vi "Receiver_Example - 2 Channel - Experiment_11.vi"() -> ()   [LabVIEW 2022 SP3]
uses:
  <vilib>/httpClient/LabVIEWHTTPClient.lvlib
panel:
  out "OutputHPCH0":i8[](array[numeric])
  out "HP - CH0 3":dbl format="%#_4g"
  out "HP - CH0 2":dbl format="%#_4g"
  out "BER 16QAM":dbl
  out "LP - CH0":dbl format="%#_4g"
  in  "url 2":string="http://Cobot280-02.local:5000"
  out "Numeric":i32
  out "HP - CH0":dbl format="%#_4g"
  in  "url":string="http://Cobot280-01.local:5000"
  out "x = 0?":bool
  out "iterationsIM":dbl
  in  "State":i32
  in  "Counter":dbl
  in  "Tab Control 3":enum32{"OFDM - 4QAM", "16QAM"}(tab)
  in  "Switch mode":bool
  in  "Tab Control":T1(tab)
  in  "USRP ControledParameters":T2={"Active Antenna"="RX2", "Gain (dB)"=10.0, "Carrier Frequency"=2400000000.0, "IQ Rate"=2000000.0, "Active channels"="0,1"} {"IQ Rate" format="%#_6p"; "Carrier Frequency" format="%#_6p"; "Gain (dB)" format="%#_6f"}
  in  "Device selection":refnum<k15>="RIO0"
  in  "Trigger level":dbl=0.005 format="%f"
  out "CH0":T3
  out "CH1":T3
  out "SIG valid? - CH1":bool
  out "SIG valid? - CH0":bool
  out "Frequency offset - CH1":dbl
  out "Frequency offset - CH0":dbl
  out "Coerced Parameters":T4={"IQ Rate"=100000.0, "Carrier  Freq."=100000.0, "Gain"=0.0} {"Gain" format="%#_6f"; "Carrier  Freq." format="%#_6p"; "IQ Rate" format="%#_6p"}
  out "Error out":errorcluster
  in  "Expected message LP - CH0":string="Non Critical Data\nNon Critical Data\nNon Critical Data\nNon Critical Data\nNon Critical Data"
  in  "Expected message - CH1":string="Critical Dataaaaa\nCritical Dataaaaa\nCritical Dataaaaa\nCritical Dataaaaa\nCritical Dataaaaa"
  out "Expected message LP Detected CH0":string="Non Critical Data\nNon Critical Data\nNon Critical Data\nNon Critical Data\nNon Critical Data"
  out "Expected message HP Detected CH1":string="Non Critical Data\nNon Critical Data\nNon Critical Data\nNon Critical Data\nNon Critical Data"
  in  "Boolean":bool
  in  "Boolean 3":bool
  out "Expected message HP Detected CH0":string="Non Critical Data\nNon Critical Data\nNon Critical Data\nNon Critical Data\nNon Critical Data"
  in  "Expected message HP - CH0":string="Critical Dataaaaa\nCritical Dataaaaa\nCritical Dataaaaa\nCritical Dataaaaa\nCritical Dataaaaa"
  in  "Boolean 2":bool
  out "Inst. BER HP - CH0":dbl format="%#_4g"
  out "Acc. BER HP - CH0":dbl format="%#_4g"
  out "Acum. Err HP - CH0":dbl
  out "No. Bits HP - CH0":dbl
  out "Acc. BER LP - CH0":dbl format="%#_4g"
  out "Inst. BER - CH1":dbl format="%#_4g"
  out "Inst. BER LP - CH0":dbl format="%#_4g"
  out "No. Bits - CH1":dbl
  out "No. Bits LP - CH0":dbl
  out "Acum. Err - CH1":dbl
  out "Acum. Err LP - CH0":dbl
  in  "Record BER":bool
  in  "Refresh Button":bool
  out "Acc. BER - CH1":dbl format="%#_4g"
  in  "High-Power Window Size":dbl=15.0 format="%#_6p"
  in  "Low-Power Window Size - CH0":dbl=15.0 format="%#_6p"
  in  "Threshold":dbl=10.0
  in  "Channel":bool
  in  "Expected message HP - CH0 2":string="Critical Dataaaaa\nCritical Dataaaaa\nCritical Dataaaaa\nCritical Dataaaaa\nCritical Dataaaaa\nNon Critical Data\nNon Critical Data\nNon Critical Data\nNon Critical Data\nNon Critical Data"
  in  "Tab Control 2":enum32{"1 Channel", "2 Channel"}(tab)
  in  "Save data 1 channel":bool
  out "Constellation Map 1 Channel":cdb[](graph)
  out "Low-Power BER - 1 Channel":dbl(graph)
  out "High-Power BER - 1 Channel":dbl(graph)
  out "High-Power Decoded message - 1 Channel":string
  out "Low-Power Decoded message - 1 Channel":string
  in  "Color Box":u32(colorbox)=11025761
  in  "Color Box 2":u32(colorbox)=7377308
  out "Low-Power Decoded message - CH0":string
  out "Decoded message - CH1":string
  out "Constellation Map 2 Channel":cluster{"Constellation":cdb[]}[](graph)
  out "Low-Power BER - CH0":dbl(graph)
  out "High-Power BER":T5(graph)
  out "High-Power Decoded message - CH0":string
  out "CH1 2":bool
  out "CH0 2":bool
  in  "Save data 2 channels":bool
  in  "Save data":bool
  out "Expected message  HP  Detected 2":string="Critical Dataaaaa\nCritical Dataaaaa\nCritical Dataaaaa\nCritical Dataaaaa\nCritical Dataaaaa"
  in  "Boolean 4":bool
  in  "High-Power Window Size 2":dbl=15.0 format="%#_6p"
  out "High-Power Instantaneous BER Graph 2":u8(slide) scale=0.0..100.0
  out "High-Power BER Graph 2":dbl(graph)
  out "No. Bits HP 2":dbl
  out "Acc. BER  HP 2":dbl format="%#_4g"
  out "Acum. Err HP 2":dbl
  out "Inst. BER HP 2":dbl format="%#_4g"
  in  "Expected message 2 HP 2":string="Critical Dataaaaa\nCritical Dataaaaa\nCritical Dataaaaa\nCritical Dataaaaa\nCritical Dataaaaa"
  out "High-Power Decoded Message 2":string
  in  "Record BER 2":bool
  out "Constellation Map 2":cdb[](graph)
  out "Frequency offset 2":dbl
  out "SIG valid? 2":bool
  in  "Refresh Button 2":bool
  out "Error out 2":errorcluster
  in  "error in (no error)":errorcluster
  # "OFDM Superposition Coded Receiver"
  # "Superposition coded\n(criticality-aware)"
  # "Single stream\n(criticality-agnostic)"
  # "1 Channel"
  # "2 Channel"
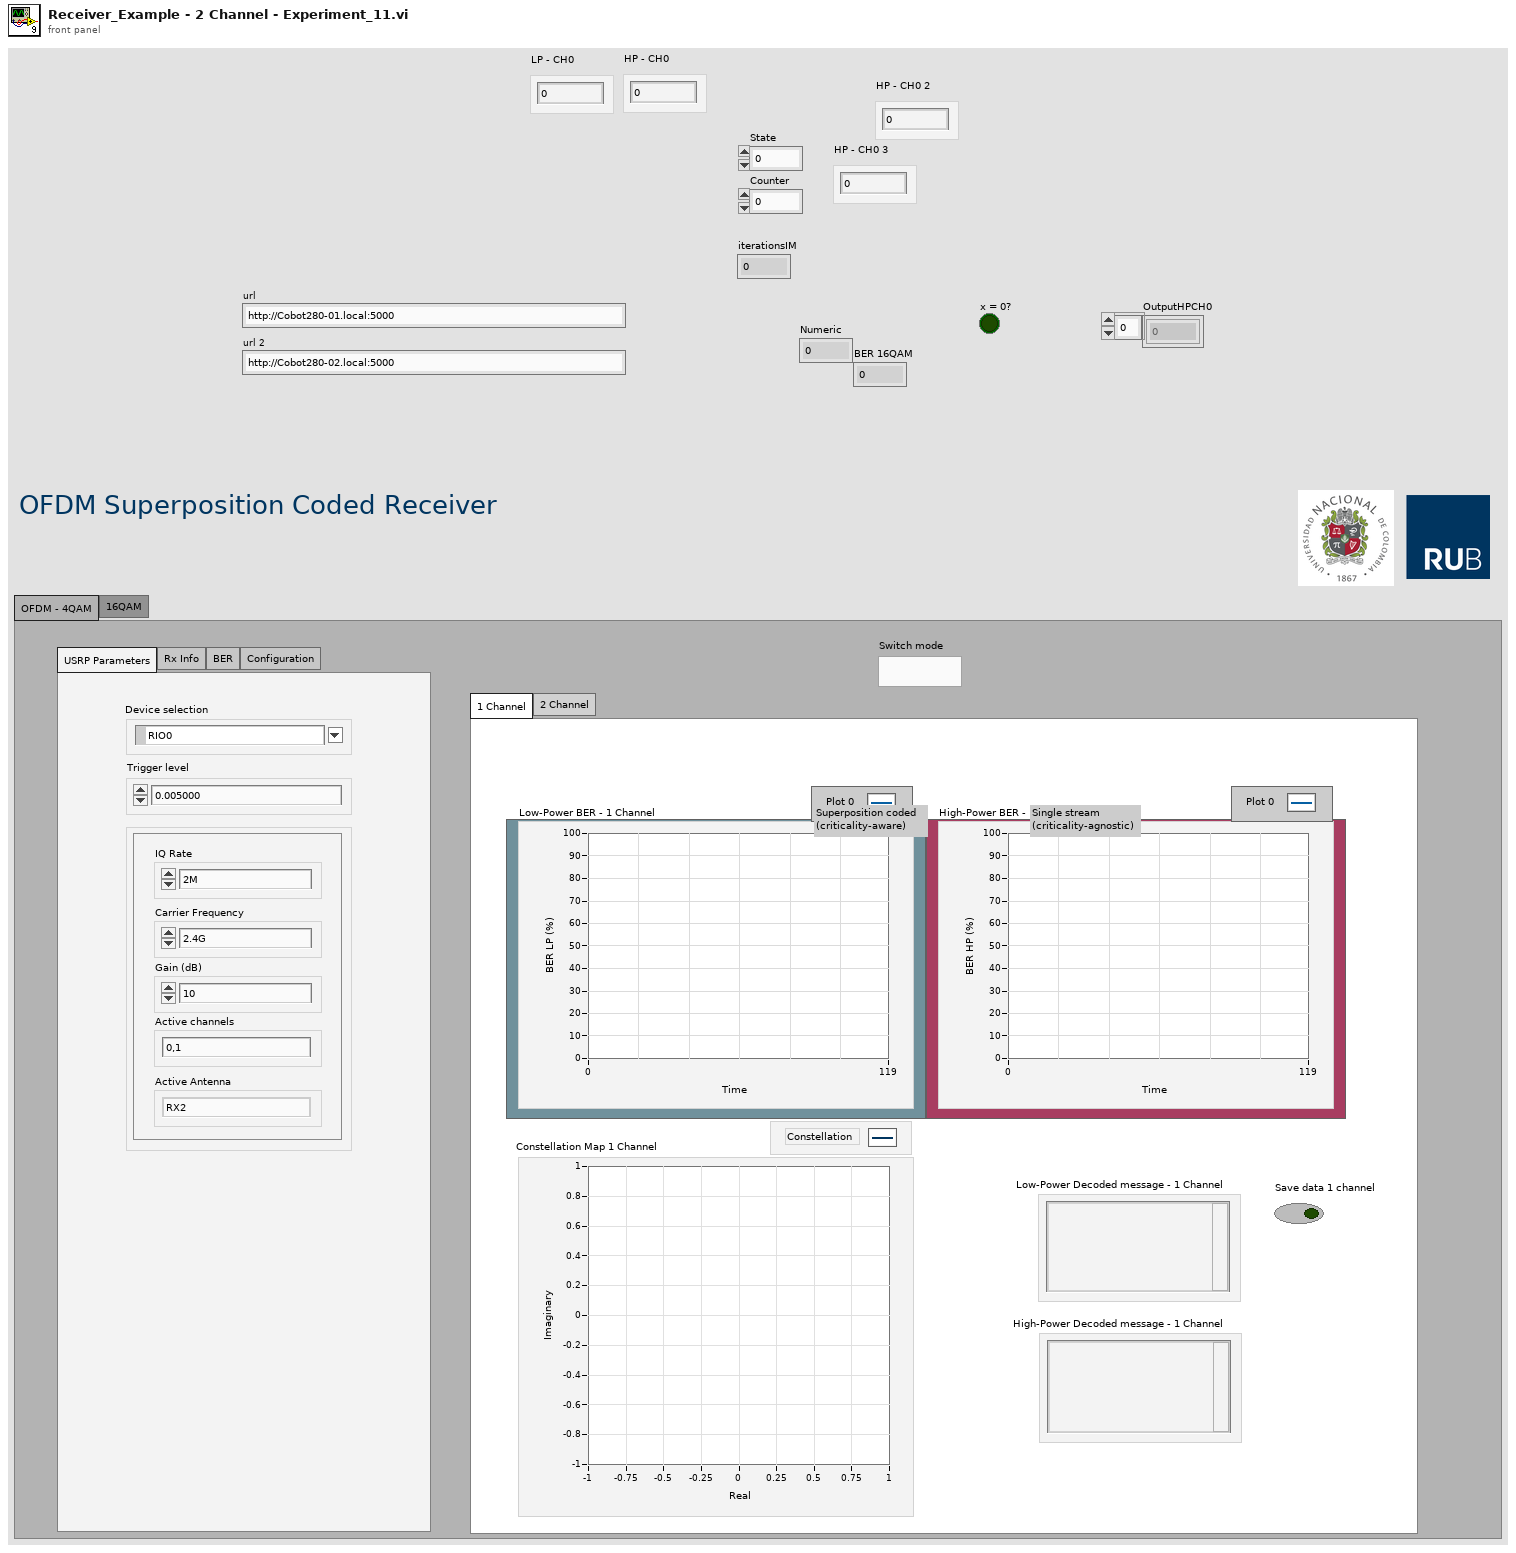
[diagram p1: front panel]
types:
  T1 = enum32{"USRP Parameters", "Rx Info", "BER", "Configuration"}
  T2 = cluster{"Active Antenna":string, "Gain (dB)":dbl, "Carrier Frequency":dbl, "IQ Rate":dbl, "Active channels":string}
  T3 = cluster{"Modulation type":enum16{"QPSK(4QAM)", "64QAM", "16QAM", "BPSK"}, "BCC rate (k/n)":enum16{"1/2", "2/3", "3/4"}}
  T4 = cluster{"IQ Rate":dbl, "Carrier  Freq.":dbl, "Gain":dbl}
  T5 = cluster{"Graph Instantaneous BER":dbl, "Graph Instantaneous BER":dbl, "Inst. BER - CH1":dbl}
  T6 = enum16{"open", "replace", "create", "open or create", "replace or create", "replace or create with confirmation"}
  T7 = cluster{"coerced IQ rate":dbl, "coerced carrier frequency":dbl, "coerced gain":dbl}
  T8 = cluster{"Graph Instantaneous BER":dbl, "Graph Instantaneous BER":dbl, "Graph Instantaneous BER":dbl}
  T9 = typedef "LabVIEWHTTPClient.lvlib/ClientHandle.ctl" = refnum<k1>
  T10 = typedef "angle_speed_def.ctl" = cluster{"degrees":dbl[], "speed":i32}
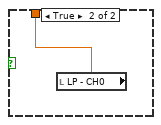
[diagram p2: hidden frame]
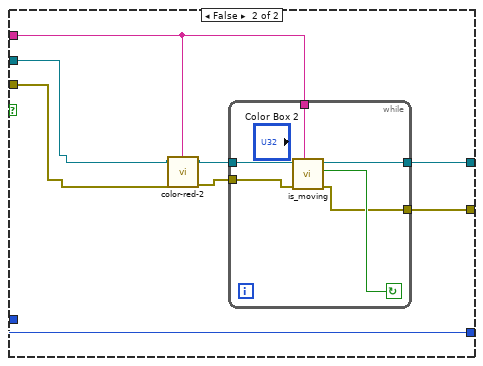
[diagram p3: hidden frame]
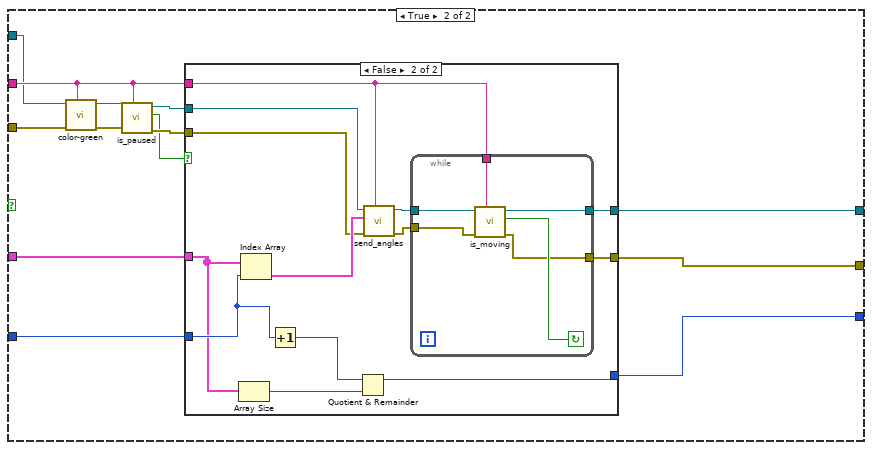
[diagram p4: hidden frame]
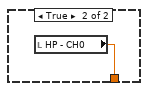
[diagram p6: hidden frame]
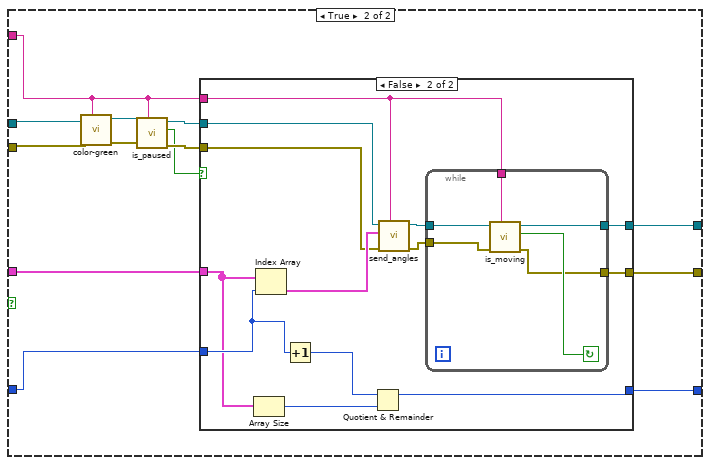
[diagram p8: hidden frame]
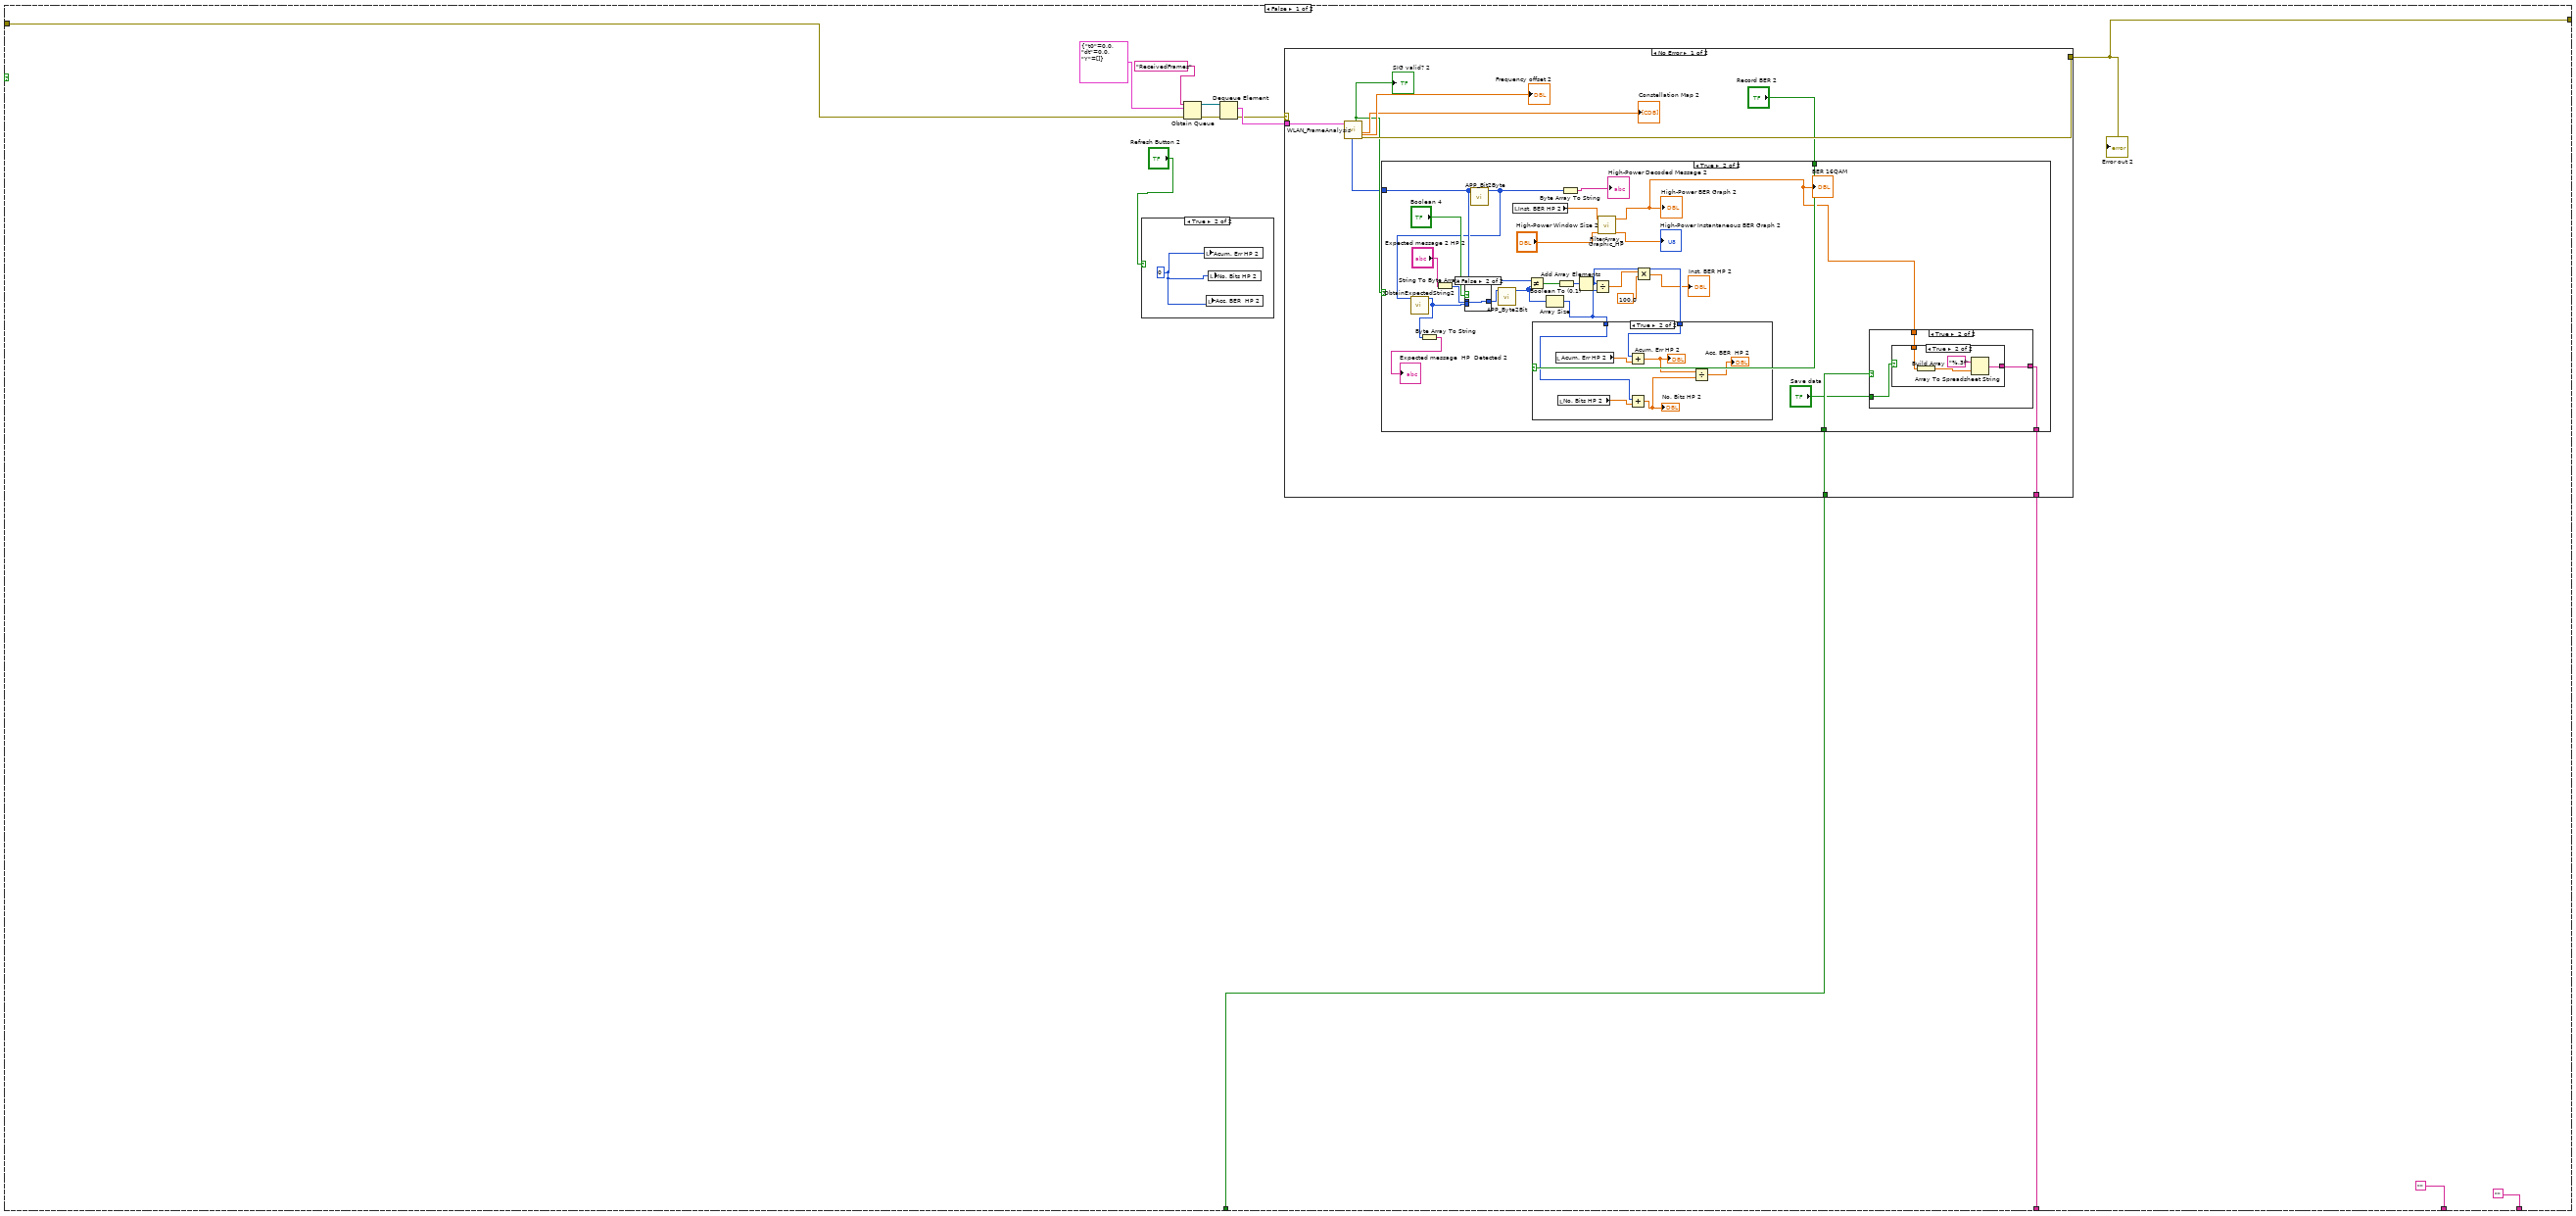
[diagram p10: hidden frame]
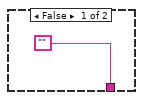
[diagram p12: hidden frame]
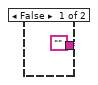
[diagram p13: hidden frame]
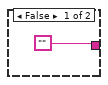
[diagram p14: hidden frame]
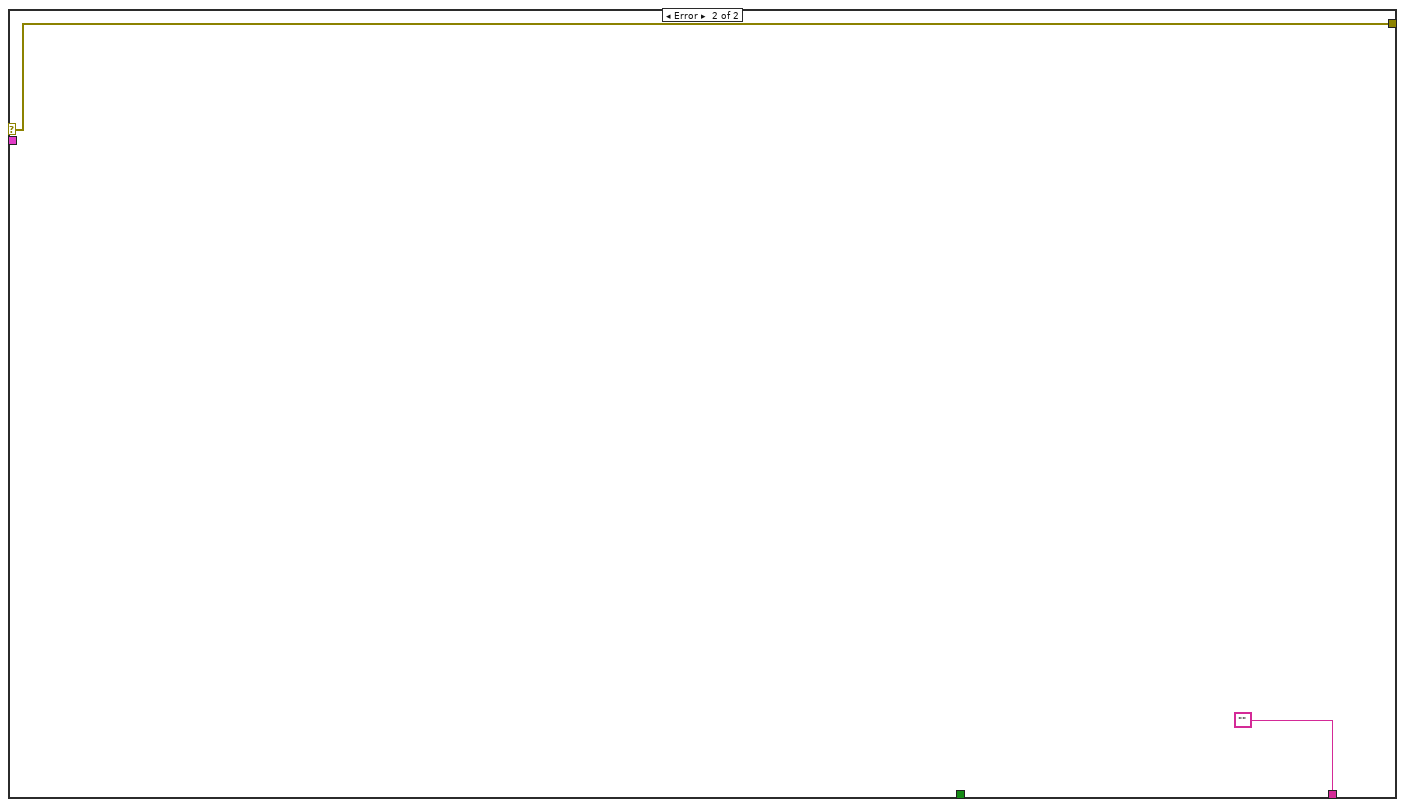
[diagram p17: hidden frame]
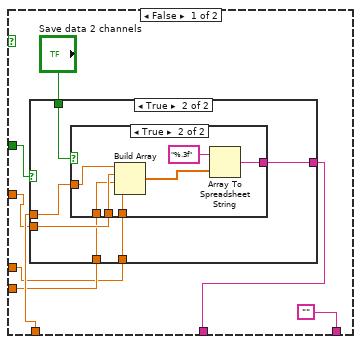
[diagram p19: hidden frame]
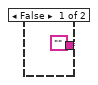
[diagram p20: hidden frame]
diagram:
  w23 = path "C:/Users/DKS/Desktop/Experiment/23_11_2023_with_graphs/12.10.2023/Supercoded Receiver with BER 12.10.2023/OFDM-Framework-LabVIEW-master/data"
  w45 = 0
  n1 = Build Path(base path=w23, name or relative path=path "data_OneChannel.txt" ("default name")) -> (appended path=w33:path)
  n2 = Build Path(base path=w23, name or relative path=path "data_16QAM.txt" ("default name")) -> (appended path=w43:path)
  n3 = Build Path(base path=w23, name or relative path=path "data_TwoChannels.txt" ("default name")) -> (appended path=w28:path)
  n4 = Delete(path (use dialog)=w33) -> (deleted path=w32:path)  [unwired: 4 in, 2 out]
  n5 = Delete(path (use dialog)=w43) -> (deleted path=w42:path)  [unwired: 4 in, 2 out]
  n6 = call "USRP_RXInit.vi"("device names"="Device selection", "USRP ControledParameters"="USRP ControledParameters", "error in (no error)"="error in (no error)") -> ("session handle out"=w48:refnum<k15>, "USRP CoercedParamters"=→"Coerced Parameters":T7, "error out"=w51:errorcluster)  [unwired: 5 in]
  n7 = Delete(path (use dialog)=w28) -> (deleted path=w27:path)  [unwired: 4 in, 2 out]
  n8 = Open/Create/Replace File(file path (use dialog)=w32, operation (0:open)=T6."create", access (0:read/write)=enum16{"read/write", "read-only", "write-only"}."write-only") -> (refnum out=w20:refnum<file>, error out=w19:errorcluster)  [unwired: 1 in, 3 out]
  n9 = Open/Create/Replace File(file path (use dialog)=w42, operation (0:open)=T6."create", access (0:read/write)=enum16{"read/write", "read-only", "write-only"}."write-only") -> (refnum out=w36:refnum<file>, error out=w37:errorcluster)  [unwired: 1 in, 3 out]
  n10 = Open/Create/Replace File(file path (use dialog)=w27, operation (0:open)=T6."create", access (0:read/write)=enum16{"read/write", "read-only", "write-only"}."write-only") -> (refnum out=w18:refnum<file>, error out=w17:errorcluster)  [unwired: 1 in, 3 out]
  n11 = call "WLAN_FrameCapture - 2 Channels.vi"("error in (no error)"=w51, "Trigger level"="Trigger level", "session handle"=w48) -> ()  [unwired: 8 in]
  n12 = while {
    tunnel: w51 -> [w77]
    tunnel: [w76] -> w49
    shift-right: [w71] -> w35
    shift-left: w37 -> [w69]
    shift-right: [w70] -> w34
    shift-left: w36 -> [w68]
    shift-right: [w65] -> w16
    shift-left: w20 -> [w66]
    shift-right: [w63] -> w15
    shift-left: w19 -> [w64]
    shift-right: [w59] -> w14
    shift-left: w18 -> [w62]
    shift-right: [w60] -> w13
    shift-left: w17 -> [w61]
    i -> [w56]
    stop <- FALSE stop-if-true
    n13 = Not(x="Switch mode") -> ()  [unwired: 1 out]
    n14 = Quotient & Remainder(x=w56, y=1) -> (x-y*floor(x/y)=w73:i32)  [unwired: 1 out]
    n15 = Equal To 0?(x=w73) -> (x = 0?=w72:bool)
    "x = 0?" <- w72
    n16 = case shown="True" TRUE {
      tunnel: w77 -> [w83 w164]
      tunnel: [w82 w163] -> w76
      tunnel: w72 -> [w81 w158]
      tunnel: [w80 ""] -> w67
      tunnel: ["" w157] -> w58
      tunnel: ["" w155] -> w57
      frame False {
        n17 = case shown="True" "Refresh Button 2" {
          frame False {
          }
          frame True {
            w91 = 0
            n18 = local write "Acum. Err HP 2"(w91) -> ()
            n19 = local write "Acc. BER  HP 2"(w91) -> ()
            n20 = local write "No. Bits HP 2"(w91) -> ()
          }
        }
        n21 = Obtain Queue(name (unnamed)="ReceivedFrames", element data type=cluster{"t0":dbl, "dt":dbl, "Y":cdb[]} {"t0"=0.0, "dt"=0.0, "Y"=[]} ("data"), error in (no error)=w83) -> (queue out=w84:refnum<queue>, error out=w87:errorcluster)  [unwired: 2 in, 1 out]
        n22 = Dequeue Element(queue=w84, error in (no error)=w87) -> (element=w86:cluster{"t0":dbl, "dt":dbl, "Y":cdb[]}, error out=w85:errorcluster)  [unwired: 1 in, 2 out]
        n23 = case shown="No Error" w85 {
          selector: w85 -> [_ w146]
          tunnel: w86 -> [w99 _]
          tunnel: [w100 w146] -> w82
          tunnel: w81 -> [w93 _]
          tunnel: [w92 ""] -> w80
          frame No Error {
            n24 = call "WLAN_FrameAnalysis.vi"("input cluster"=w99) -> ("error out"=w100:errorcluster, "Constellation"=→"Constellation Map 2":cdb[], "Frequency offset"=→"Frequency offset 2":dbl, "SIG valid?"=w95:bool, "outputbitsHP"=w94:i8[])  [unwired: 4 in, 2 out]
            "SIG valid? 2" <- w95
            n25 = case shown="True" w95 {
              tunnel: "Record BER 2" -> [_ w120]
              tunnel: w94 -> [_ w115]
              tunnel: w93 -> [_ w105]
              tunnel: ["" w103] -> w92
              frame False {
              }
              frame True {
                n26 = String To Byte Array(string="Expected message 2 HP 2") -> (unsigned byte array=w113:u8[])
                n27 = call "APP_Bit2Byte.vi"("input bit stream"=w115) -> ("output byte stream"=w109:u8[])  [unwired: 10 in]
                n28 = call "ObtainExpectedString2.vi"("Array"=w109) -> ("detectedMessage"=w111:i8[])  [unwired: 9 in]
                n29 = Byte Array To String(unsigned byte array=w111) -> (string=→"Expected message  HP  Detected 2":string)
                n30 = case shown="False" "Boolean 4" {
                  tunnel: [w136 w137] -> w114
                  tunnel: w113 -> [_ w137]
                  tunnel: w111 -> [w136 _]
                  frame True {
                  }
                  frame False {
                  }
                }
                n31 = call "APP_Byte2Bit.vi"("input byte stream"=w114) -> ("output bit stream"=w116:i8[])  [unwired: 10 in]
                n32 = local read "Inst. BER HP 2"() -> (w119:dbl)
                n33 = Not Equal?(x=w115, y=w116) -> (x != y?=w124:bool[])
                n34 = Array Size(array=w116) -> (size(s)=w121:i32)
                n35 = Boolean To (0,1)(Boolean=w124) -> (0, 1=w123:i16[])
                n36 = Byte Array To String(unsigned byte array=w109) -> (string=→"High-Power Decoded Message 2":string)
                n37 = Add Array Elements(numeric array=w123) -> (sum=w122:i16)
                n38 = case shown="True" w120 {
                  tunnel: w122 -> [_ w143]
                  tunnel: w121 -> [_ w138]
                  frame False {
                  }
                  frame True {
                    n39 = local read "Acum. Err HP 2"() -> (w144:dbl)
                    n40 = local read "No. Bits HP 2"() -> (w140:dbl)
                    n41 = Add(x=w143, y=w144) -> (x+y=w142:dbl)
                    "Acum. Err HP 2" <- w142
                    n42 = Add(x=w138, y=w140) -> (x+y=w139:dbl)
                    "No. Bits HP 2" <- w139
                    n43 = Divide(x=w142, y=w139) -> (x/y=→"Acc. BER  HP 2":dbl)
                  }
                }
                n44 = Divide(x=w122, y=w121) -> (x/y=w108:dbl)
                n45 = call "FilterArray_Graphic_HP.vi"("Window Size"="High-Power Window Size 2", "Instantaneous BER"=w119) -> ("Slide Bar"=→"High-Power Instantaneous BER Graph 2":dbl, "Graph Instantaneous BER"=w102:dbl)  [unwired: 4 in]
                "High-Power BER Graph 2" <- w102
                "BER 16QAM" <- w102
                n46 = Multiply(x=w108, y=100.0) -> (x*y=→"Inst. BER HP 2":dbl)
                n47 = case shown="True" w105 {
                  tunnel: ["" w130] -> w103
                  tunnel: w102 -> [_ w129]
                  tunnel: "Save data" -> [_ w128]
                  frame False {
                  }
                  frame True {
                    n48 = case shown="True" w128 {
                      tunnel: ["" w133] -> w130
                      tunnel: w129 -> [_ w132]
                      frame False {
                      }
                      frame True {
                        n49 = Build Array(w132) -> (w135:dbl[])
                        n50 = Array To Spreadsheet String(array=w135, 3:"%.3f") -> (spreadsheet string=w133:string)  [unwired: 1 out]
                      }
                    }
                  }
                }
              }
            }
          }
          frame Error {
          }
        }
        "Error out 2" <- w82
      }
      frame True {
        w200 = cluster{"t0":dbl, "dt":dbl, "Y":cdb[]} {"t0"=0.0, "dt"=0.0, "Y"=[]} ("data")
        n51 = Obtain Queue(name (unnamed)="ReceivedFrames", element data type=w200, error in (no error)=w164) -> (queue out=w165:refnum<queue>, error out=w167:errorcluster)  [unwired: 2 in, 1 out]
        n52 = Obtain Queue(name (unnamed)="ReceivedFrames_1", element data type=w200, error in (no error)=w164) -> (queue out=w169:refnum<queue>, error out=w170:errorcluster)  [unwired: 2 in, 1 out]
        n53 = Dequeue Element(queue=w165, error in (no error)=w167) -> (element=w166:cluster{"t0":dbl, "dt":dbl, "Y":cdb[]}, error out=w173:errorcluster)  [unwired: 1 in, 2 out]
        n54 = Dequeue Element(queue=w169, error in (no error)=w170) -> (element=w175:cluster{"t0":dbl, "dt":dbl, "Y":cdb[]}, error out=w179:errorcluster)  [unwired: 1 in, 2 out]
        n55 = Not(x="Channel") -> (.not. x?=w159:bool)
        n56 = Merge Errors(w173, w179) -> (w172:errorcluster)
        n57 = case shown="No Error" w172 {
          tunnel: w166 -> [w349 _]
          tunnel: w172 -> [_ w449]
          tunnel: w173 -> [w346 _]
          tunnel: [w345 dbl[] []] -> w191
          tunnel: [w344 w449] -> w176
          tunnel: "Record BER" -> [w343 _]
          tunnel: "Record BER" -> [w342 _]
          tunnel: w159 -> [w341 _]
          frame No Error {
            n58 = local read "Switch mode"() -> (w340:bool)
            n59 = call "WLAN_FrameAnalysis.vi"("error in (no error)"=w346, "input cluster"=w349) -> ("error out"=w344:errorcluster, "Constellation"=w345:cdb[], "Modulation parameter"=w350:T3, "output bits"=w351:i8[], "Frequency offset"=→"Frequency offset - CH0":dbl, "SIG valid?"=w347:bool, "outputbitsHP"=w348:i8[])  [unwired: 3 in]
            "SIG valid? - CH0" <- w347
            n60 = Not(x=w340) -> (.not. x?=w339:bool)
            n61 = case shown="True" w347 {
              tunnel: w351 -> [_ w401]
              tunnel: w350 -> [_ w424]
              tunnel: w342 -> [_ w420]
              tunnel: w341 -> [_ w404]
              tunnel: w339 -> [_ w402]
              frame False {
              }
              frame True {
                n62 = case shown="False" w402 {
                  tunnel: w401 -> [_ w434]
                  tunnel: [w432 w434] -> w403
                  frame False {
                    n63 = local read "OutputHPCH0"() -> (w431:i8[])
                    n64 = Array Size(array=w431) -> (size(s)=w430:i32)
                    n65 = Divide(x=w430, y=2) -> (x/y=w427:dbl)
                    n66 = Add(x=4.0, y=w427) -> (x+y=w429:dbl)
                    n67 = Subtract(x=w427, y=5.0) -> (x-y=w425:dbl)
                    n68 = Array Subset(array=w431, index=w429, length=w425) -> (w432:i8[])
                  }
                  frame True {
                  }
                }
                n69 = String To Byte Array(string="Expected message LP - CH0") -> (unsigned byte array=w413:u8[])
                n70 = call "APP_Bit2Byte.vi"("input bit stream"=w403) -> ("output byte stream"=w412:u8[])  [unwired: 10 in]
                n71 = call "ObtainExpectedString.vi"("Array"=w412) -> ("detectedMessage"=w409:i8[])  [unwired: 9 in]
                n72 = Byte Array To String(unsigned byte array=w409) -> (string=→"Expected message LP Detected CH0":string)
                n73 = case shown="False" "Boolean" {
                  tunnel: [w439 w440] -> w415
                  tunnel: w413 -> [_ w440]
                  tunnel: w409 -> [w439 _]
                  frame True {
                  }
                  frame False {
                  }
                }
                n74 = call "APP_Byte2Bit.vi"("input byte stream"=w415) -> ("output bit stream"=w414:i8[])  [unwired: 10 in]
                n75 = Not Equal?(x=w401, y=w414) -> (x != y?=w422:bool[])
                n76 = Array Size(array=w414) -> (size(s)=w419:i32)
                n77 = Boolean To (0,1)(Boolean=w422) -> (0, 1=w423:i16[])
                n78 = Add Array Elements(numeric array=w423) -> (sum=w418:i16)
                n79 = case shown="True" w420 {
                  tunnel: w419 -> [_ w446]
                  tunnel: w418 -> [_ w444]
                  frame False {
                  }
                  frame True {
                    n80 = local read "Acum. Err LP - CH0"() -> (w445:dbl)
                    n81 = local read "No. Bits LP - CH0"() -> (w447:dbl)
                    n82 = Add(x=w446, y=w447) -> (x+y=w443:dbl)
                    n83 = Add(x=w444, y=w445) -> (x+y=w442:dbl)
                    "Acum. Err LP - CH0" <- w442
                    n84 = local write "No. Bits LP - CH0"(w443) -> ()
                    n85 = Divide(x=w442, y=w443) -> (x/y=→"Acc. BER LP - CH0":dbl)
                  }
                }
                n86 = Divide(x=w418, y=w419) -> (x/y=w417:dbl)
                n87 = Multiply(x=w417, y=100.0) -> (x*y=→"Inst. BER LP - CH0":dbl)
                n88 = Byte Array To String(unsigned byte array=w412) -> (string=w407:string)
                n89 = case shown="True" w404 {
                  tunnel: w407 -> [w436 w438]
                  tunnel: ["" ("string") w438] -> w406
                  tunnel: [w436 "" ("string")] -> w405
                  frame False {
                  }
                  frame True {
                  }
                }
                "Low-Power Decoded message - CH0" <- w405
                "Low-Power Decoded message - 1 Channel" <- w406
                "CH0" <- w424
              }
            }
            n90 = case shown="True" w347 {
              tunnel: w348 -> [_ w354]
              tunnel: w343 -> [_ w372]
              tunnel: w341 -> [_ w359]
              tunnel: w339 -> [_ w357]
              frame False {
              }
              frame True {
                n91 = String To Byte Array(string="Expected message HP - CH0") -> (unsigned byte array=w356:u8[])
                n92 = case shown="False" w357 {
                  tunnel: w354 -> [w383 w387]
                  tunnel: [w384 w387] -> w358
                  tunnel: [w376 w386] -> w353
                  tunnel: w356 -> [_ w386]
                  frame False {
                    n93 = Array Size(array=w383) -> (size(s)=w380:i32)
                    n94 = Divide(x=w380, y=2) -> (x/y=w379:dbl)
                    n95 = Subtract(x=w379, y=5) -> (x-y=w381:dbl)
                    n96 = Array Subset(array=w383, index=0, length=w381) -> (w384:i8[])
                    n97 = String To Byte Array(string="Expected message HP - CH0 2") -> (unsigned byte array=w376:u8[])
                  }
                  frame True {
                  }
                }
                n98 = call "APP_Byte2Bit.vi"("input byte stream"=w353) -> ("output bit stream"=w355:i8[])  [unwired: 10 in]
                n99 = Not Equal?(x=w354, y=w355) -> (x != y?=w374:bool[])
                n100 = Array Size(array=w355) -> (size(s)=w371:i32)
                n101 = Boolean To (0,1)(Boolean=w374) -> (0, 1=w375:i16[])
                n102 = Add Array Elements(numeric array=w375) -> (sum=w370:i16)
                n103 = case shown="True" w372 {
                  tunnel: w371 -> [_ w399]
                  tunnel: w370 -> [_ w397]
                  frame False {
                  }
                  frame True {
                    n104 = local read "Acum. Err HP - CH0"() -> (w398:dbl)
                    n105 = local read "No. Bits HP - CH0"() -> (w400:dbl)
                    n106 = Add(x=w399, y=w400) -> (x+y=w396:dbl)
                    n107 = local write "No. Bits HP - CH0"(w396) -> ()
                    n108 = Add(x=w397, y=w398) -> (x+y=w395:dbl)
                    "Acum. Err HP - CH0" <- w395
                    n109 = Divide(x=w395, y=w396) -> (x/y=→"Acc. BER HP - CH0":dbl)
                  }
                }
                n110 = Divide(x=w370, y=w371) -> (x/y=w369:dbl)
                n111 = call "APP_Bit2Byte.vi"("input bit stream"=w358) -> ("output byte stream"=w365:u8[])  [unwired: 10 in]
                n112 = call "ObtainExpectedString2.vi"("Array"=w365) -> ("detectedMessage"=w364:i8[])  [unwired: 9 in]
                n113 = Byte Array To String(unsigned byte array=w364) -> (string=→"Expected message HP Detected CH0":string)
                n114 = case shown="False" "Boolean 2" {
                  tunnel: [w392 w393] -> _
                  tunnel: w356 -> [_ w393]
                  tunnel: w364 -> [w392 _]
                  frame True {
                  }
                  frame False {
                  }
                }
                n115 = Multiply(x=w369, y=100.0) -> (x*y=→"Inst. BER HP - CH0":dbl)
                n116 = Byte Array To String(unsigned byte array=w365) -> (string=w360:string)
                n117 = case shown="False" w359 {
                  tunnel: w360 -> [w389 w391]
                  tunnel: ["" ("string") w391] -> w361
                  tunnel: [w389 "" ("string")] -> w362
                  frame False {
                  }
                  frame True {
                  }
                }
                "High-Power Decoded message - CH0" <- w362
                "High-Power Decoded message - 1 Channel" <- w361
                "OutputHPCH0" <- w354
              }
            }
          }
          frame Error {
          }
        }
        n118 = case shown="No Error" w179 {
          tunnel: w175 -> [w299 _]
          tunnel: "Record BER" -> [w297 _]
          tunnel: [w296 w338] -> w177
          tunnel: [w295 dbl[] []] -> w178
          tunnel: w179 -> [w294 w338]
          tunnel: w159 -> [w293 _]
          frame No Error {
            n119 = call "WLAN_FrameAnalysis.vi"("error in (no error)"=w294, "input cluster"=w299) -> ("error out"=w296:errorcluster, "Constellation"=w295:cdb[], "Modulation parameter"=w302:T3, "Frequency offset"=→"Frequency offset - CH1":dbl, "SIG valid?"=w298:bool, "outputbitsHP"=w300:i8[])  [unwired: 3 in, 1 out]
            "SIG valid? - CH1" <- w298
            n120 = case shown="True" "Refresh Button" {
              frame False {
              }
              frame True {
                w304 = 0
                n121 = local write "Acum. Err HP - CH0"(w304) -> ()
                n122 = local write "Acc. BER HP - CH0"(w304) -> ()
                n123 = local write "Acum. Err LP - CH0"(w304) -> ()
                n124 = local write "No. Bits LP - CH0"(w304) -> ()
                n125 = local write "No. Bits HP - CH0"(w304) -> ()
                n126 = local write "Acc. BER LP - CH0"(w304) -> ()
                n127 = local write "Acum. Err - CH1"(w304) -> ()
                n128 = local write "No. Bits - CH1"(w304) -> ()
                n129 = local write "Acc. BER - CH1"(w304) -> ()
              }
            }
            n130 = case shown="True" w298 {
              tunnel: w300 -> [_ w311]
              tunnel: w302 -> [_ w325]
              tunnel: w297 -> [_ w308]
              tunnel: w293 -> [_ w305]
              frame False {
              }
              frame True {
                n131 = call "APP_Bit2Byte.vi"("input bit stream"=w311) -> ("output byte stream"=w314:u8[])  [unwired: 10 in]
                n132 = call "ObtainExpectedString3.vi"("Array"=w314) -> ("detectedMessage"=w313:i8[])  [unwired: 9 in]
                n133 = Byte Array To String(unsigned byte array=w314) -> (string=w306:string)
                n134 = String To Byte Array(string="Expected message - CH1") -> (unsigned byte array=w315:u8[])
                n135 = Byte Array To String(unsigned byte array=w313) -> (string=→"Expected message HP Detected CH1":string)
                n136 = case shown="False" "Boolean 3" {
                  tunnel: [w328 w329] -> w317
                  tunnel: w315 -> [_ w329]
                  tunnel: w313 -> [w328 _]
                  frame True {
                  }
                  frame False {
                  }
                }
                n137 = call "APP_Byte2Bit.vi"("input byte stream"=w317) -> ("output bit stream"=w316:i8[])  [unwired: 10 in]
                n138 = Not Equal?(x=w311, y=w316) -> (x != y?=w323:bool[])
                n139 = Array Size(array=w316) -> (size(s)=w321:i32)
                n140 = Boolean To (0,1)(Boolean=w323) -> (0, 1=w324:i16[])
                n141 = Add Array Elements(numeric array=w324) -> (sum=w320:i16)
                n142 = case shown="True" w308 {
                  tunnel: w321 -> [_ w335]
                  tunnel: w320 -> [_ w333]
                  frame False {
                  }
                  frame True {
                    n143 = local read "No. Bits - CH1"() -> (w336:dbl)
                    n144 = local read "Acum. Err - CH1"() -> (w334:dbl)
                    n145 = Add(x=w335, y=w336) -> (x+y=w332:dbl)
                    n146 = Add(x=w333, y=w334) -> (x+y=w331:dbl)
                    "Acum. Err - CH1" <- w331
                    n147 = local write "No. Bits - CH1"(w332) -> ()
                    n148 = Divide(x=w331, y=w332) -> (x/y=→"Acc. BER - CH1":dbl)
                  }
                }
                n149 = case shown="True" w305 {
                  tunnel: w306 -> [w326 _]
                  tunnel: [w326 "" ("string")] -> w307
                  frame False {
                  }
                  frame True {
                  }
                }
                "Decoded message - CH1" <- w307
                n150 = Divide(x=w320, y=w321) -> (x/y=w318:dbl)
                n151 = Multiply(x=w318, y=100.0) -> (x*y=→"Inst. BER - CH1":dbl)
                "CH1" <- w325
              }
            }
          }
          frame Error {
          }
        }
        n152 = local read "Inst. BER HP - CH0"() -> (w196:dbl)
        n153 = local read "Inst. BER - CH1"() -> (w186:dbl)
        n154 = Bundle("Constellation"=w191) -> (w190:cluster{"Constellation":cdb[]})  [unwired: 1 in]
        n155 = Bundle("Constellation"=w178) -> (w174:cluster{"Constellation":cdb[]})  [unwired: 1 in]
        n156 = local read "Inst. BER LP - CH0"() -> (w161:dbl)
        n157 = Merge Errors(w176, w177) -> (w163:errorcluster)
        "Error out" <- w163
        n158 = Build Array(w190, w174) -> (w193:cluster{"Constellation":cdb[]}[])
        n159 = call "FilterArray_Graphic_CH1.vi"("Window Size"="High-Power Window Size", "Instantaneous BER"=w186) -> ("Graph Instantaneous BER"=w156:dbl)  [unwired: 4 in, 1 out]
        n160 = call "FilterArray_Graphic_HP.vi"("Window Size"="High-Power Window Size", "Instantaneous BER"=w196) -> ("Graph Instantaneous BER"=w153:dbl)  [unwired: 4 in, 1 out]
        "HP - CH0" <- w153
        n161 = case shown="0, Default" "State" {
          tunnel: "Counter" -> [w261 w281]
          tunnel: [w268 w284] -> w182
          tunnel: "Counter" -> [w256 w274]
          tunnel: [w265 w283] -> w183
          tunnel: [w263 w282] -> w154
          tunnel: w153 -> [w262 w279]
          tunnel: w156 -> [w260 w280]
          tunnel: 10.0 ("y") -> [w259 w275]
          frame 0, Default {
            n162 = Greater?(x=w262, y=10.0) -> (0:w269:bool)
            n163 = Equal?(x=w256, y=w259) -> (x = y?=w264:bool)
            n164 = Add(x=w261, y=1.0) -> (x+y=w271:dbl)
            n165 = Greater?(x=w256, y=w259) -> (0:w258:bool)
            n166 = Select(t=w271, s=w269, f=0.0) -> (s? t:f=w268:dbl)
            n167 = Select(t=w260, s=w264, f=w262) -> (s? t:f=w263:dbl)
            n168 = Select(t=1.0, s=w264, f=0.0) -> (s? t:f=w265:dbl)
            n169 = Select(t=0.0, s=w258, f=w256) -> (s? t:f=w255:dbl)
            n170 = local write "Counter"(w255) -> ()
          }
          frame 1 {
            n171 = Less?(x=w279, y=10.0) -> (x < y?=w285:bool)
            n172 = Greater?(x=w274, y=w275) -> (0:w277:bool)
            n173 = Equal?(x=w274, y=w275) -> (x = y?=w287:bool)
            n174 = Add(x=w281, y=1.0) -> (x+y=w291:dbl)
            n175 = Select(t=w291, s=w285, f=0.0) -> (s? t:f=w284:dbl)
            n176 = Select(t=0.0, s=w277, f=w274) -> (s? t:f=w278:dbl)
            n177 = local write "Counter"(w278) -> ()
            n178 = Select(t=w279, s=w287, f=w280) -> (s? t:f=w282:dbl)
            n179 = Select(t=0.0, s=w287, f=1.0) -> (s? t:f=w283:dbl)
          }
        }
        n180 = call "FilterArray_Graphic_LP.vi"("Window Size"="Low-Power Window Size - CH0", "Instantaneous BER"=w161) -> ("Graph Instantaneous BER"=w152:dbl)  [unwired: 4 in, 1 out]
        "LP - CH0" <- w152
        n181 = case shown="True" w159 {
          tunnel: [cdb[] [] ("Constellation") w254] -> w192
          tunnel: w191 -> [_ w254]
          tunnel: w193 -> [w252 _]
          tunnel: [w252 cluster{"Constellation":cdb[]}[] []] -> w194
          frame False {
          }
          frame True {
          }
        }
        "Constellation Map 2 Channel" <- w194
        "Constellation Map 1 Channel" <- w192
        n182 = local read "Switch mode"() -> (w151:bool)
        n183 = case shown="False" w159 {
          tunnel: w152 -> [w244 w246]
          tunnel: [nan ("Graph Instantaneous BER") w246] -> w148
          tunnel: [w244 nan ("Graph Instantaneous BER")] -> w149
          frame False {
          }
          frame True {
          }
        }
        "Low-Power BER - CH0" <- w149
        n184 = Bundle("Graph Instantaneous BER"=w153, "Graph Instantaneous BER"=w156, "Graph Instantaneous BER"=w154) -> (w198:T8)  [unwired: 1 in]
        n185 = Equal To 0?(x="State") -> (x = 0?=w189:bool)
        "CH0 2" <- w189
        n186 = Not(x=w151) -> (.not. x?=w150:bool)
        n187 = Not(x=w189) -> (.not. x?=→"CH1 2":bool)
        n188 = case shown="False" w159 {
          tunnel: w153 -> [_ w250]
          tunnel: [nan w250] -> w197
          tunnel: w198 -> [w248 _]
          tunnel: [w248 T8 {"Graph Instantaneous BER"=nan, "Graph Instantaneous BER"=nan, "Graph Instantaneous BER"=nan}] -> w199
          frame False {
          }
          frame True {
          }
        }
        "High-Power BER" <- w199
        "High-Power BER - 1 Channel" <- w197
        n189 = case shown="False" w150 {
          tunnel: w148 -> [_ w202]
          tunnel: [w201 w202] -> w147
          frame False {
            n190 = local read "HP - CH0"() -> (w201:dbl)
          }
          frame True {
          }
        }
        "Low-Power BER - 1 Channel" <- w147
        n191 = local write "Counter"(w182) -> ()
        n192 = local write "State"(w183) -> ()
        n193 = case shown="True" w159 {
          tunnel: w152 -> [w207 w231]
          tunnel: w153 -> [w206 w230]
          tunnel: w158 -> [w209 w229]
          tunnel: ["" w227] -> w157
          tunnel: w156 -> [w205 _]
          tunnel: w154 -> [w204 _]
          tunnel: [w203 ""] -> w155
          frame False {
            n194 = case shown="True" w209 {
              tunnel: ["" w217] -> w203
              tunnel: w207 -> [_ w215]
              tunnel: w206 -> [_ w216]
              tunnel: "Save data 2 channels" -> [_ w214]
              tunnel: w205 -> [_ w213]
              tunnel: w204 -> [_ w212]
              frame False {
              }
              frame True {
                n195 = case shown="True" w214 {
                  tunnel: ["" w223] -> w217
                  tunnel: w215 -> [_ w222]
                  tunnel: w216 -> [_ w221]
                  tunnel: w213 -> [_ w220]
                  tunnel: w212 -> [_ w219]
                  frame False {
                  }
                  frame True {
                    n196 = Build Array(w222, w221, w220, w219) -> (w225:dbl[])
                    n197 = Array To Spreadsheet String(array=w225, 3:"%.3f") -> (spreadsheet string=w223:string)  [unwired: 1 out]
                  }
                }
              }
            }
          }
          frame True {
            n198 = case shown="True" w229 {
              tunnel: ["" w236] -> w227
              tunnel: w231 -> [_ w234]
              tunnel: w230 -> [_ w235]
              tunnel: "Save data 1 channel" -> [_ w233]
              frame False {
              }
              frame True {
                n199 = case shown="True" w233 {
                  tunnel: ["" w240] -> w236
                  tunnel: w234 -> [_ w239]
                  tunnel: w235 -> [_ w238]
                  frame False {
                  }
                  frame True {
                    n200 = Build Array(w239, w238) -> (w242:dbl[])
                    n201 = Array To Spreadsheet String(array=w242, 3:"%.3f") -> (spreadsheet string=w240:string)  [unwired: 1 out]
                  }
                }
              }
            }
          }
        }
      }
    }
    n202 = Write to Text File(file (use dialog)=w62, text=w57, error in=w61) -> (refnum out=w59:refnum<file>, error out=w60:errorcluster)  [unwired: 1 in, 1 out]
    n203 = Write to Text File(file (use dialog)=w68, text=w67, error in=w69) -> (refnum out=w70:refnum<file>, error out=w71:errorcluster)  [unwired: 1 in, 1 out]
    n204 = Write to Text File(file (use dialog)=w66, text=w58, error in=w64) -> (refnum out=w65:refnum<file>, error out=w63:errorcluster)  [unwired: 1 in, 1 out]
    "Numeric" <- w56
  }
  n205 = call <vilib>:"OpenHandle.vi"() -> ("client handle out"=w7:T9, "error out"=w8:errorcluster)  [unwired: 14 in]
  n206 = call "wave.vi"() -> ("sequenz"=w9:T10[])  [unwired: 11 in]
  n207 = call <vilib>:"OpenHandle.vi"() -> ("client handle out"=w3:T9, "error out"=w2:errorcluster)  [unwired: 14 in]
  n208 = while {
    shift-right: [w459] -> _
    shift-left: 0 -> [w460]
    tunnel: w9 -> [w458]
    tunnel: w2 -> [w457]
    tunnel: w3 -> [w456]
    tunnel: [w455] -> w6
    tunnel: [w454] -> w4
    tunnel: "Threshold" -> [w453]
    stop <- FALSE stop-if-true
    n209 = local read "Switch mode"() -> (w451:bool)
    n210 = Not(x=w451) -> (.not. x?=w450:bool)
    n211 = case shown="False" w450 {
      tunnel: [w465 w466] -> w452
      frame False {
        n212 = local read "HP - CH0"() -> (w465:dbl)
      }
      frame True {
        n213 = local read "LP - CH0"() -> (w466:dbl)
      }
    }
    n214 = Wait (ms)(milliseconds to wait=u32 300) -> ()  [unwired: 1 out]
    n215 = Less?(x=w452, y=w453) -> (x < y?=w462:bool)
    n216 = case shown="False" w462 {
      tunnel: "url 2" -> [w471 w501]
      tunnel: w460 -> [w473 w500]
      tunnel: [w472 w499] -> w459
      tunnel: w458 -> [_ w498]
      tunnel: w457 -> [w468 w497]
      tunnel: w456 -> [w467 w496]
      tunnel: [w470 w495] -> w455
      tunnel: [w469 w494] -> w454
      frame False {
        n217 = call "is_paused.vi"("url"=w471, "error in (no error)"=w468, "client handle"=w467) -> ("error out"=w475:errorcluster, "paused"=w474:bool, "client handle out"=w476:T9)  [unwired: 6 in]
        n218 = case shown="True" w474 {
          tunnel: w471 -> [_ w482]
          tunnel: w475 -> [w478 w484]
          tunnel: w476 -> [w479 w483]
          tunnel: [w479 w487] -> w470
          tunnel: [w478 w486] -> w469
          tunnel: w473 -> [w477 w485]
          tunnel: [w477 w485] -> w472
          frame True {
          }
          frame False {
            n219 = call "color-red-2.vi"("url"=w482, "error in (no error)"=w484, "client handle"=w483) -> ("error out"=w480:errorcluster, "client handle out"=w481:T9)  [unwired: 7 in]
            n220 = while {
              tunnel: w482 -> [w493]
              tunnel: w481 -> [w492]
              tunnel: w480 -> [w491]
              tunnel: [w489] -> w487
              tunnel: [w488] -> w486
              stop <- w490 continue-if-true
              n221 = call "is_moving.vi"("string"=w493, "error in (no error)"=w491, "client handle"=w492) -> ("error out"=w488:errorcluster, "moving"=w490:bool, "client handle out"=w489:T9)  [unwired: 6 in]
            }
          }
        }
      }
      frame True {
        n222 = call "color-green.vi"("url"=w501, "error in (no error)"=w497, "client handle"=w496) -> ("error out"=w503:errorcluster, "client handle out"=w502:T9)  [unwired: 7 in]
        n223 = call "is_paused.vi"("url"=w501, "error in (no error)"=w503, "client handle"=w502) -> ("error out"=w505:errorcluster, "paused"=w504:bool, "client handle out"=w506:T9)  [unwired: 6 in]
        n224 = case shown="False" w504 {
          tunnel: w498 -> [_ w514]
          tunnel: w500 -> [w507 w516]
          tunnel: w501 -> [_ w519]
          tunnel: w505 -> [w508 w521]
          tunnel: w506 -> [w509 w520]
          tunnel: [w507 w512] -> w499
          tunnel: [w509 w511] -> w495
          tunnel: [w508 w510] -> w494
          frame True {
          }
          frame False {
            n225 = Array Size(array=w514) -> (size(s)=w513:i32)
            n226 = Index Array(array=w514, index=w516) -> (element=w522:T10)
            n227 = Increment(x=w516) -> (x+1=w515:i32)
            n228 = Quotient & Remainder(x=w515, y=w513) -> (x-y*floor(x/y)=w512:i32)  [unwired: 1 out]
            n229 = call "send_angles.vi"("url"=w519, "error in (no error)"=w521, "angles and speed"=w522, "client handle"=w520) -> ("error out"=w517:errorcluster, "client handle out"=w518:T9)  [unwired: 6 in]
            n230 = while {
              tunnel: w519 -> [w528]
              tunnel: w518 -> [w527]
              tunnel: w517 -> [w526]
              tunnel: [w524] -> w511
              tunnel: [w523] -> w510
              stop <- w525 continue-if-true
              n231 = call "is_moving.vi"("string"=w528, "error in (no error)"=w526, "client handle"=w527) -> ("error out"=w523:errorcluster, "moving"=w525:bool, "client handle out"=w524:T9)  [unwired: 6 in]
            }
          }
        }
      }
    }
  }
  n232 = while {
    tunnel: w9 -> [w542]
    tunnel: w8 -> [w541]
    tunnel: w7 -> [w540]
    tunnel: [w539] -> w12
    tunnel: [w538] -> w5
    shift-right: [w536] -> _
    shift-left: 0 -> [w537]
    tunnel: "Threshold" -> [w531]
    stop <- FALSE stop-if-true
    n233 = local read "Switch mode"() -> (w529:bool)
    n234 = case shown="False" w529 {
      tunnel: [w543 w544] -> w530
      frame False {
        n235 = local read "HP - CH0"() -> (w543:dbl)
      }
      frame True {
        n236 = local read "HP - CH0"() -> (w544:dbl)
      }
    }
    n237 = Wait (ms)(milliseconds to wait=u32 300) -> ()  [unwired: 1 out]
    n238 = Less?(x=w530, y=w531) -> (x < y?=w534:bool)
    n239 = case shown="False" w534 {
      tunnel: w542 -> [_ w582]
      tunnel: w537 -> [w549 w573]
      tunnel: w541 -> [w550 w574]
      tunnel: w540 -> [w551 w575]
      tunnel: [w547 w581] -> w539
      tunnel: [w546 w580] -> w538
      tunnel: [w548 w578] -> w536
      tunnel: "url" -> [w545 w572]
      frame False {
        n240 = call "is_paused.vi"("url"=w545, "error in (no error)"=w550, "client handle"=w551) -> ("error out"=w553:errorcluster, "paused"=w552:bool, "client handle out"=w554:T9)  [unwired: 6 in]
        n241 = case shown="False" w552 {
          tunnel: w545 -> [_ w558]
          tunnel: w553 -> [w556 w560]
          tunnel: w554 -> [w557 w559]
          tunnel: [w557 w565] -> w547
          tunnel: [w556 w564] -> w546
          tunnel: w549 -> [w555 w563]
          tunnel: [w555 w563] -> w548
          frame True {
          }
          frame False {
            n242 = call "color-red.vi"("url"=w558, "error in (no error)"=w560, "client handle"=w559) -> ("error out"=w561:errorcluster, "client handle out"=w562:T9)  [unwired: 7 in]
            n243 = while {
              tunnel: w558 -> [w571]
              tunnel: w562 -> [w570]
              tunnel: w561 -> [w569]
              tunnel: [w567] -> w565
              tunnel: [w566] -> w564
              stop <- w568 continue-if-true
              n244 = call "is_moving.vi"("string"=w571, "error in (no error)"=w569, "client handle"=w570) -> ("error out"=w566:errorcluster, "moving"=w568:bool, "client handle out"=w567:T9)  [unwired: 6 in]
            }
          }
        }
      }
      frame True {
        n245 = call "color-green.vi"("url"=w572, "error in (no error)"=w574, "client handle"=w575) -> ("error out"=w577:errorcluster, "client handle out"=w576:T9)  [unwired: 7 in]
        n246 = call "is_paused.vi"("url"=w572, "error in (no error)"=w577, "client handle"=w576) -> ("error out"=w583:errorcluster, "paused"=w579:bool, "client handle out"=w584:T9)  [unwired: 6 in]
        n247 = case shown="False" w579 {
          tunnel: w582 -> [_ w592]
          tunnel: w573 -> [w585 w594]
          tunnel: w572 -> [_ w597]
          tunnel: w583 -> [w586 w599]
          tunnel: w584 -> [w587 w598]
          tunnel: [w585 w590] -> w578
          tunnel: [w587 w589] -> w581
          tunnel: [w586 w588] -> w580
          frame True {
          }
          frame False {
            n248 = Array Size(array=w592) -> (size(s)=w591:i32)
            n249 = Index Array(array=w592, index=w594) -> (element=w600:T10)
            n250 = Increment(x=w594) -> (x+1=w593:i32)
            n251 = Quotient & Remainder(x=w593, y=w591) -> (x-y*floor(x/y)=w590:i32)  [unwired: 1 out]
            n252 = call "send_angles.vi"("url"=w597, "error in (no error)"=w599, "angles and speed"=w600, "client handle"=w598) -> ("error out"=w595:errorcluster, "client handle out"=w596:T9)  [unwired: 6 in]
            n253 = while {
              tunnel: w597 -> [w606]
              tunnel: w596 -> [w605]
              tunnel: w595 -> [w604]
              tunnel: [w602] -> w589
              tunnel: [w601] -> w588
              stop <- w603 continue-if-true
              n254 = call "is_moving.vi"("string"=w606, "error in (no error)"=w604, "client handle"=w605) -> ("error out"=w601:errorcluster, "moving"=w603:bool, "client handle out"=w602:T9)  [unwired: 6 in]
            }
          }
        }
      }
    }
  }
  n255 = call <vilib>:"CloseHandle.vi"("client handle"=w6, "error in (no error)"=w4) -> ()  [unwired: 13 in, 1 out]
  n256 = call <vilib>:"CloseHandle.vi"("client handle"=w12, "error in (no error)"=w5) -> ()  [unwired: 13 in, 1 out]
  n257 = Close File(refnum=w34, error in=w35) -> (error out=w38:errorcluster)  [unwired: 1 out]
  n258 = Close File(refnum=w16, error in=w15) -> (error out=w22:errorcluster)  [unwired: 1 out]
  n259 = Close File(refnum=w14, error in=w13) -> (error out=w21:errorcluster)  [unwired: 1 out]
  n260 = local read "iterationsIM"() -> (→"iterationsIM":dbl)
  n261 = call <vilib>:"Simple Error Handler.vi"("error in (no error)"=w38) -> ()  [unwired: 1 in, 8 out]
  n262 = call <vilib>:"Simple Error Handler.vi"("error in (no error)"=w22) -> ()  [unwired: 1 in, 8 out]
  n263 = call <vilib>:"Simple Error Handler.vi"("error in (no error)"=w21) -> ()  [unwired: 1 in, 8 out]
  n264 = call <instrlib>:"niUSRP Close Session.vi"("session handle"=w48, "error in (no error)"=w49) -> ()  [unwired: 13 in, 1 out]
  "No. Bits LP - CH0" <- w45
  "No. Bits - CH1" <- w45
  "No. Bits HP - CH0" <- w45
